vi "Init Resolve.vi"(11 "Map in":refnum<class "Map.lvclass">) -> (1 "New Map out":refnum<class "Map.lvclass">)   [LabVIEW 2020, in "SquareBattle.lvlib" / "Map.lvclass"]
uses:
  Map.lvclass
  Map.lvclass/Map.ctl
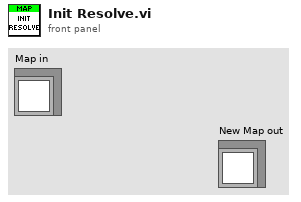
[diagram p1: front panel]
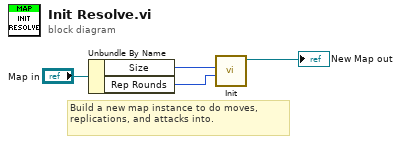
[diagram p0: block diagram]
diagram:
  # "Build a new map instance to do moves, replications, and attacks into."
  n1 = Unbundle By Name("Map in") -> ("Size"=w3:i32, "Rep Rounds"=w2:u32)
  n2 = call "Init.vi"("Replication Rounds"=w2, "Size"=w3) -> ("Map out"=→"New Map out":refnum<class "Map.lvclass">)  [unwired: 8 in, 1 out]
